vi "simple_math.vi"(2 "Y":dbl, 3 "X":dbl, 4 "Irons Range":dbl, 5 "Wind":dbl(slide) scale=0.0..360.0) -> (0 "Y out":dbl, 1 "X out":dbl)   [LabVIEW 2013]
panel:
  out "slope tackline":dbl
  out "slope wind":dbl
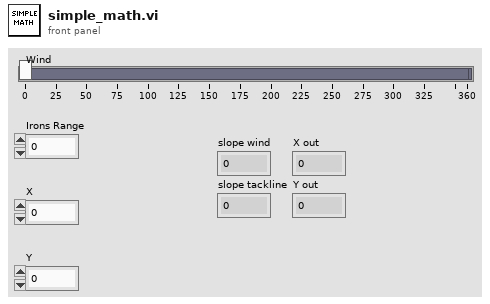
[diagram p1: front panel]
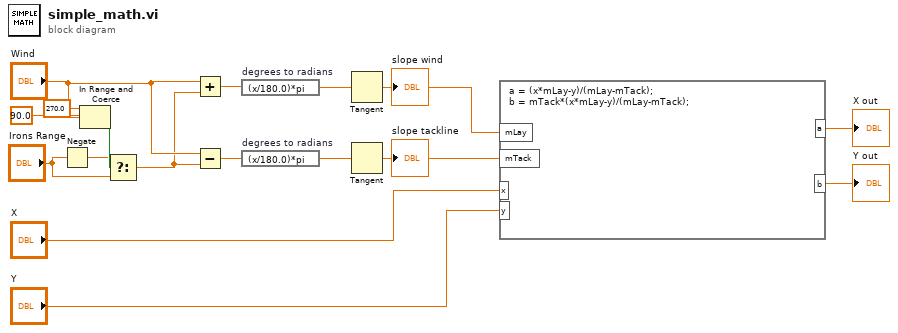
[diagram p0: block diagram]
diagram:
  n1 = Negate(x="Irons Range") -> (-x=w2:dbl)
  n2 = In Range and Coerce(upper limit=270.0, x="Wind", lower limit=90.0) -> (In Range?=w4:bool)  [unwired: 1 out]
  n3 = Select(t=w2, s=w4, f="Irons Range") -> (s? t:f=w3:dbl)
  n4 = Add(x="Wind", y=w3) -> (x+y=w17:dbl)
  n5 = Subtract(x="Wind", y=w3) -> (x-y=w14:dbl)
  n6 = expression code="(x/180.0)*pi" "degrees to radians"(w17) -> (w16:dbl)
  n7 = expression code="(x/180.0)*pi" "degrees to radians"(w14) -> (w15:dbl)
  n8 = Tangent(1:w16) -> (0:w13:dbl)
  "slope wind" <- w13
  n9 = Tangent(1:w15) -> (0:w12:dbl)
  "slope tackline" <- w12
  n10 = formula code="a = (x*mLay-y)/(mLay-mTack);\nb = mTack*(x*mLay-y)/(mLay-mTack);"("mLay"=w13, "mTack"=w12, "x"="X", "y"="Y") -> ("a"=→"X out":dbl, "b"=→"Y out":dbl)
